vi "Register Path.vi"(8 "error in (no error)":errorcluster, 10 "Path":path, 11 "Key":variant) -> (0 "error out":errorcluster, 2 "Value Unchanged?":bool, 3 "Key Already Included?":bool)   [LabVIEW 2021, in "Path Utilities.lvlib"]
doc: "Register a Path associated with a Key.\nIf the key is already registered, this function replaces the original Path of the corresponding Key with the new Path value.\n\nNo error is returned."
uses:
  Path Utilities.lvlib
  TypeDefs/FGV State - Path Registration.ctl
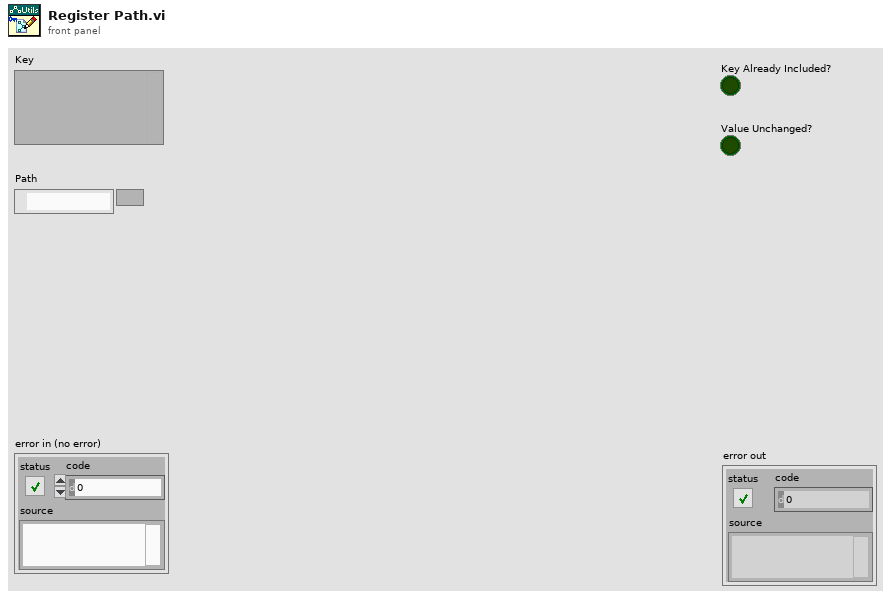
[diagram p1: front panel]
types:
  T1 = typedef "Path Utilities.lvlib/FGV State - Path Registration.ctl" = enum16{"Get Path", "Register Path", "Unregister Path"}
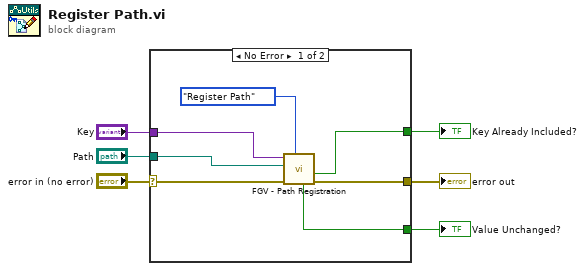
[diagram p0: block diagram]
diagram:
  n1 = case shown="No Error" "error in (no error)" {
    selector: "error in (no error)" -> [w13 w14]
    tunnel: [w12 w14] -> w5
    tunnel: "Path" -> [w11 _]
    tunnel: "Key" -> [w10 _]
    tunnel: [w8 _] -> w2
    tunnel: [w7 _] -> w1
    frame No Error {
      n2 = call "FGV - Path Registration.vi"("FGV State"=FGV_State_-_Path_Registration."Register Path", "error in (no error)"=w13, "Path"=w11, "Key"=w10) -> ("error out"=w12:errorcluster, "Key Already Included?"=w8:bool, "Value Unchanged?"=w7:bool)  [unwired: 3 in, 2 out]
    }
    frame Error {
    }
  }
  "error out" <- w5
  "Key Already Included?" <- w2
  "Value Unchanged?" <- w1
